vi "FPGAStartCompile.vi"(11 "viref":refnum<vi>) -> (1 "bitfile path when compile done":path)   [LabVIEW 2020, in "NI_TargetHelper.lvlib"]
uses:
  <vilib>/TargetSupport/NI_TargetHelper/NI_TargetHelper.lvlib
  <vilib>/rvi/CDR/niFpgaBuild_BuildSpecPath.ctl
  <vilib>/rvi/CDR/niFpgaBuild_BuildSpecType.ctl
  <vilib>/rvi/CDR/niFpgaBuild_Action.ctl
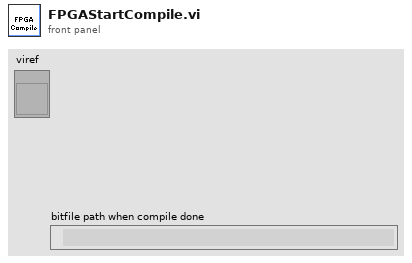
[diagram p1: front panel]
types:
  T1 = typedef "niFpgaBuild_BuildSpecType.ctl" = enum16{"Compilation", "Simulation", "VivadoProject"}
  T2 = typedef "niFpgaBuild_BuildSpecPath.ctl" = cluster{"ProjectPath":path, "TargetName":string, "BuildSpecName":string}
  T3 = typedef "niFpgaBuild_Action.ctl" = enum16{"GenerateCode", "Compile", "Download", "Run"}
  T4 = typedef "niFpgaBuild_BuildSpecProjectReferences.ctl" = cluster{"Project":refnum<vi>, "ProjectRoot":refnum<vi>, "AllTargets":refnum<vi>[], "Target":refnum<vi>, "BuildSpecificationNode":refnum<vi>, "TargetApplication":refnum<vi>}
  T5 = typedef "ItemRef.ctl" = u64
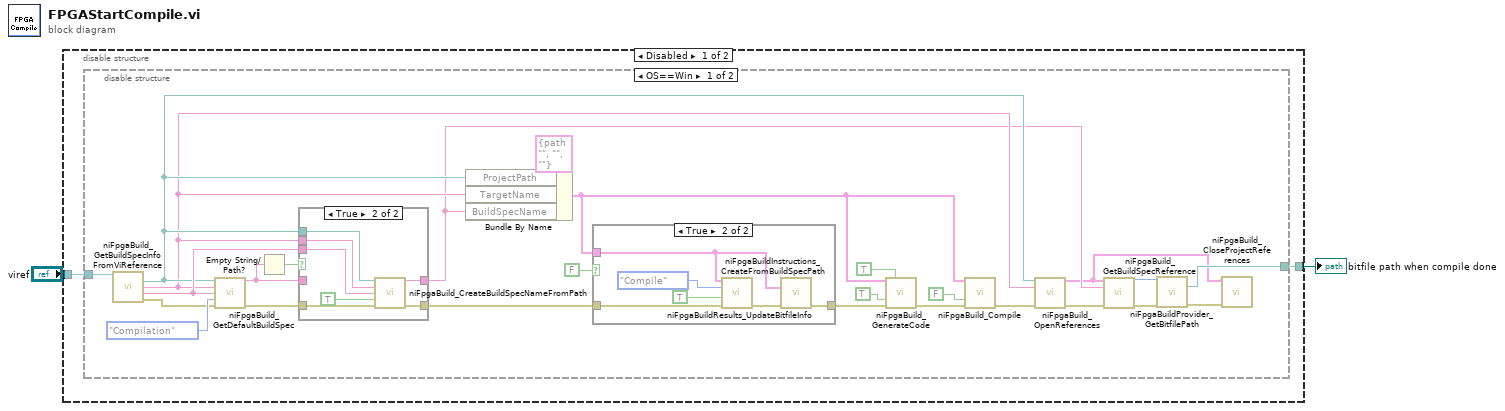
[diagram p0: block diagram]
diagram:
  n1 = disable-structure shown="Disabled" {
    disable-tunnel: "viref" -> [w4 _]
    disable-tunnel: [w3 _] -> w1
    frame Disabled {
      n2 = disable-structure shown="OS==Win" {
        disable-tunnel: w4 -> [w30 _]
        disable-tunnel: [w29 _] -> w3
        frame condition #0 {
          n3 = call <vilib>:"niFpgaBuild_GetBuildSpecInfoFromViReference.vi"("vi reference in"=w30) -> ("project path"=w13:path, "target name"=w12:string, "vi itemId"=w20:string, "error out"=w21:errorcluster)  [unwired: 10 in, 1 out]
          n4 = call <vilib>:"niFpgaBuild_GetDefaultBuildSpec.vi"("project path"=w13, "target name"=w12, "vi item ID"=w20, "buildspec type"=niFpgaBuild_BuildSpecType."Compilation", "error in (no error)"=w21) -> ("build spec name"=w27:string, "error out"=w26:errorcluster)  [unwired: 9 out]
          n5 = Empty String/Path?(string/path=w27) -> (empty?=w28:bool)
          n6 = case shown="True" w28 {
            tunnel: w27 -> [w38 _]
            tunnel: w26 -> [w39 w46]
            tunnel: [w39 w45] -> w23
            tunnel: [w38 w44] -> w10
            tunnel: w13 -> [_ w43]
            tunnel: w12 -> [_ w42]
            tunnel: w20 -> [_ w41]
            frame False {
            }
            frame True {
              n7 = call <vilib>:"niFpgaBuild_CreateBuildSpecNameFromPath.vi"("project path"=w43, "target name"=w42, "vi item ID"=w41, "make default"=TRUE, "error in (no error)"=w46) -> ("build spec name"=w44:string, "error out"=w45:errorcluster)  [unwired: 1 in, 8 out]
            }
          }
          n8 = Bundle By Name(cluster=T2 {"ProjectPath"=path "", "TargetName"="", "BuildSpecName"=""} ("build spec path"), "ProjectPath"=w13, "TargetName"=w12, "BuildSpecName"=w10) -> (w5:T2)
          n9 = case shown="True" FALSE {
            tunnel: w23 -> [w31 w35]
            tunnel: w5 -> [_ w33]
            tunnel: [w31 w32] -> w17
            frame False {
            }
            frame True {
              n10 = call <vilib>:"niFpgaBuildInstructions_CreateFromBuildSpecPath.vi"("build spec path"=w33, "action"=niFpgaBuild_Action."Compile", "display status dialogs"=TRUE, "error in (no error)"=w35) -> ("error out"=w34:errorcluster)  [unwired: 11 in]
              n11 = call <vilib>:"niFpgaBuildResults_UpdateBitfileInfo.vi"("build spec path"=w33, "error in (no error)"=w34) -> ("error out"=w32:errorcluster)  [unwired: 13 in]
            }
          }
          n12 = call <vilib>:"niFpgaBuild_GenerateCode.vi"("build spec path"=w5, "display status dialogs(T)"=TRUE, "wait until done"=TRUE, "error in (no error)"=w17) -> ("error out"=w16:errorcluster)  [unwired: 11 out]
          n13 = call <vilib>:"niFpgaBuild_Compile.vi"("build spec path"=w5, "wait until done"=FALSE, "error in (no error)"=w16) -> ("error out"=w14:errorcluster)  [unwired: 11 in, 1 out]
          n14 = call <vilib>:"niFpgaBuild_OpenReferences.vi"("project path"=w13, "target name"=w12, "error in (no error)"=w14) -> ("build spec project references"=w6:T4, "error out"=w11:errorcluster)  [unwired: 11 in]
          n15 = call <vilib>:"niFpgaBuild_GetBuildSpecReference.vi"("build spec project references"=w6, "build spec name"=w10, "error in (no error)"=w11) -> ("Item"=w8:T5, "error out"=w9:errorcluster)  [unwired: 11 in]
          n16 = call <vilib>:"niFpgaBuildProvider_GetBitfilePath.vi"("Item"=w8, "error in (no error)"=w9) -> ("bitfile path"=w29:path, "error out"=w7:errorcluster)  [unwired: 12 in]
          n17 = call <vilib>:"niFpgaBuild_CloseProjectReferences.vi"("build spec project references"=w6, "error in (no error)"=w7) -> ()  [unwired: 13 in, 1 out]
        }
        frame condition #1 (active) {
        }
      }
    }
    frame Enabled {
    }
  }
  "bitfile path when compile done" <- w1
